vi "DataLog Server Boot.vi"   [LabVIEW 2012]
doc: "Dynamically bootstrap a server VI by opening a reference and calling it. This allows this VI to be the only VI inside a built executable with all the remaining VIs, starting from the top-level server VI, located outside the executable using the very same directory layout as used during development.\n\nFor this to work, this VI must be pointed to the server VI to boot. Also, the INI file of the executable must specify a VI search path that allows vi.lib VIs and any required instr.lib VIs to be found.\n\nTo allow for a truly minimal executable, this VI does not make use of any subVIs. If it would, those particular VIs would be loaded from the executable instead of from the external source tree, thus making it impossible to replace them without rebuilding the executable."
types:
  T1 = enum32{"existing file", "new file", "new or existing file", "existing dir", "new dir", "new or existing dir", "existing file (use LLBs)", "new file (use LLBs)", "new or existing file (use LLBs)", "new or existing file or directory (use LLBs)"}
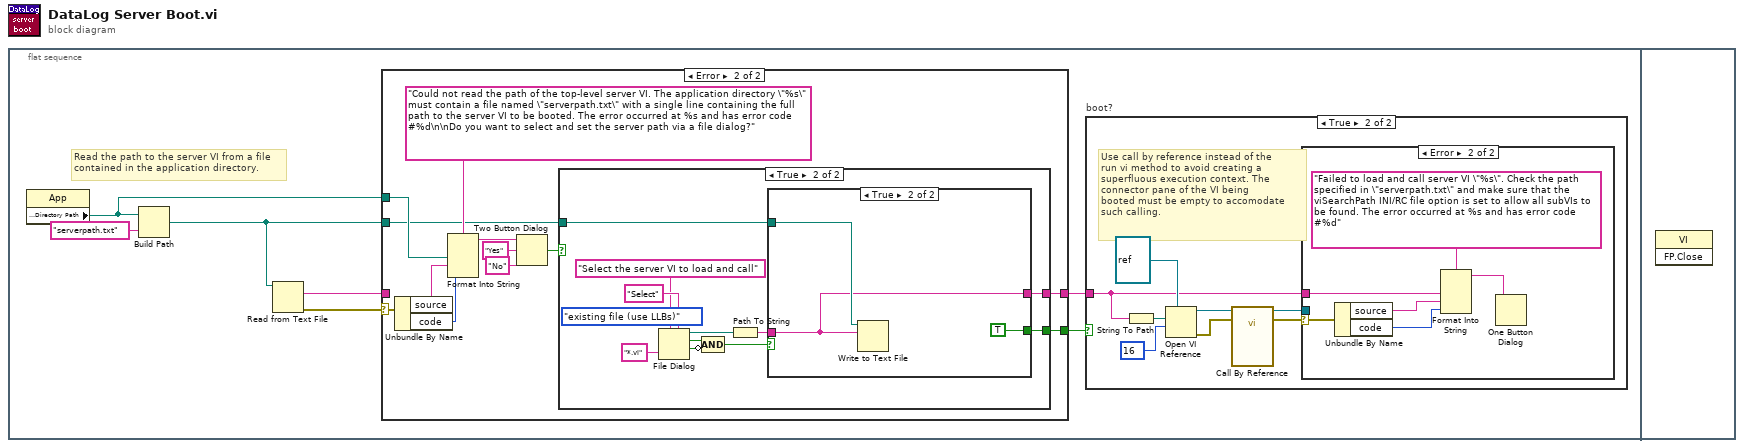
[diagram p0: block diagram]
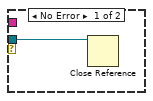
[diagram p3: hidden frame]
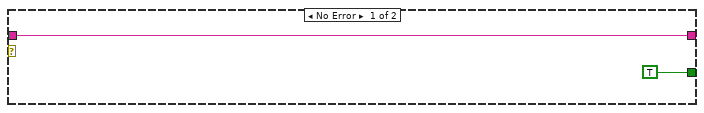
[diagram p4: hidden frame]
diagram:
  n1 = flat-sequence {
    frame #0 {
      # "Read the path to the server VI from a file\ncontained in the application directory."
      n2 = property class="App"() -> ("Application:Directory Path"=w6:path)  [unwired: 2 in, 2 out]
      n3 = Build Path(base path=w6, name or relative path="serverpath.txt") -> (appended path=w1:path)
      n4 = Read from Text File(file (use dialog)=w1) -> (text=w2:string, error out=w3:errorcluster)  [unwired: 3 in, 2 out]
      n5 = case shown="Error" w3 {
        selector: w3 -> [_ w32]
        tunnel: w2 -> [w24 _]
        tunnel: w6 -> [_ w33]
        tunnel: w1 -> [_ w28]
        tunnel: [w24 w27] -> w5
        tunnel: [TRUE w26] -> w4
        frame No Error {
        }
        frame Error {
          n6 = Unbundle By Name(w32) -> ("source"=w34:string, "code"=w25:i32)
          n7 = Format Into String(format string="Could not read the path of the top-level server VI. The application directory \"%s\" must contain a file named \"serverpath.txt\" with a single line containing the full path to the server VI to be booted. The error occurred at %s and has error code #%d\n\nDo you want to select and set the server path via a file dialog?", w33, w34, w25) -> (resulting string=w35:string)  [unwired: 2 in, 1 out]
          n8 = Two Button Dialog(message=w35, 1:"No" ("F button name (\"Cancel\")"), 2:"Yes" ("T button name (\"OK\")")) -> (T button?=w29:bool)
          n9 = case shown="True" w29 {
            tunnel: w28 -> [_ w39]
            tunnel: [_ w38] -> w27
            tunnel: [_ w37] -> w26
            frame False {
            }
            frame True {
              (unwired) T1."existing file (use LLBs)" ("select mode (2)")
              n10 = File Dialog(5:"Select" ("button label"), 6:"*.vi" ("pattern"), 7:"Select the server VI to load and call" ("prompt")) -> (1:w43:bool, 2:w44:bool, 3:w42:path)  [unwired: 4 in, 1 out]
              n11 = Compound Arithmetic op=AND(w44, invert w43) -> (w41:bool)
              n12 = Path To String(path=w42) -> (string=w40:string)
              n13 = case shown="True" w41 {
                tunnel: w40 -> [_ w48]
                tunnel: w39 -> [_ w49]
                tunnel: [_ w48] -> w38
                tunnel: [_ TRUE] -> w37
                frame False {
                }
                frame True {
                  n14 = Write to Text File(file (use dialog)=w49, text=w48) -> ()  [unwired: 2 in, 3 out]
                }
              }
            }
          }
        }
      }
      n15 = case "boot?" shown="True" w4 {
        tunnel: w5 -> [_ w9]
        frame False {
        }
        frame True {
          # "Use call by reference instead of the\nrun vi method to avoid creating a\nsuperfluous execution context. The\nconnector pane of the VI being\nbooted must be empty to accomodate\nsuch calling."
          n16 = String To Path(string=w9) -> (path=w10:path)
          n17 = Open VI Reference(type specifier VI Refnum (for type only)=refnum<vi> refnum, vi path=w10, options=16) -> (vi reference=w14:refnum<vi>, error out=w12:errorcluster)  [unwired: 3 in]
          n18 = call-by-ref "?"(reference=w14, error in=w12) -> (reference out=w11:refnum<vi>, error out=w13:errorcluster)  [unwired: 1 in]
          n19 = case shown="Error" w13 {
            selector: w13 -> [_ w21]
            tunnel: w11 -> [w16 _]
            tunnel: w9 -> [_ w18]
            frame No Error {
              n20 = Close Reference(reference=w16) -> ()  [unwired: 1 in, 1 out]
            }
            frame Error {
              n21 = Unbundle By Name(w21) -> ("source"=w19:string, "code"=w17:i32)
              n22 = Format Into String(format string="Failed to load and call server VI \"%s\". Check the path specified in \"serverpath.txt\" and make sure that the viSearchPath INI/RC file option is set to allow all subVIs to be found. The error occurred at %s and has error code #%d", w18, w19, w17) -> (resulting string=w20:string)  [unwired: 2 in, 1 out]
              n23 = One Button Dialog(message=w20) -> ()  [unwired: 1 in, 1 out]
            }
          }
        }
      }
    }
    frame #1 {
      n24 = invoke class="VI" method="FP.Close"() -> ()  [unwired: 3 in, 3 out]
    }
  }
